vi "Periodic Tasks.vi"() -> ()   [LabVIEW 2011]
doc: "This VI runs in parallel to other tasks. It can contain as many user-defined periodic loops as you need. These can carry out PID or other sorts of timed response."
uses:
  <vilib>/Rock Robotics/SystemInterfaces/Utilities/FPGA_UtilitiesLED Source.ctl
  <vilib>/Rock Robotics/SystemInterfaces/Utilities/FPGA_UtilitiesLED State.ctl
  Robot Global Data.vi
  <vilib>/Rock Robotics/WPI/Relay/WPI_RelayValue.ctl
  <vilib>/addons/control/pid/NI_PID_pid.lvlib
  <vilib>/addons/control/pid/pid.llb/PID (DBL).vi
panel:
  out "Waveform Chart 2":dynamicdata(graph)
  in  "PID gains 2":T1={"proportional gain (Kc)"=1.0, "integral time (Ti, min)"=0.01, "derivative time (Td, min)"=0.0} {"derivative time (Td, min)" format="%.3f"; "integral time (Ti, min)" format="%.3f"; "proportional gain (Kc)" format="%.3f"}
  in  "Volts per degree":dbl=0.0166666666666667
  in  "-1/1 per degree":dbl=0.05
  in  "Home Speed 2":dbl=1.0
  in  "PID Enable 2":bool
  in  "lower limit 2":dbl=0.85
  in  "upper limit 2":dbl=4.5
  out "Whole Loop Timer":u32
  out "Heading 2":u16
  out "Angular Rate":dbl
  out "Angle":dbl
  out "Direction":bool
  out "Distance":dbl
  # "Speed to move to home"
  # "Target Tracking"
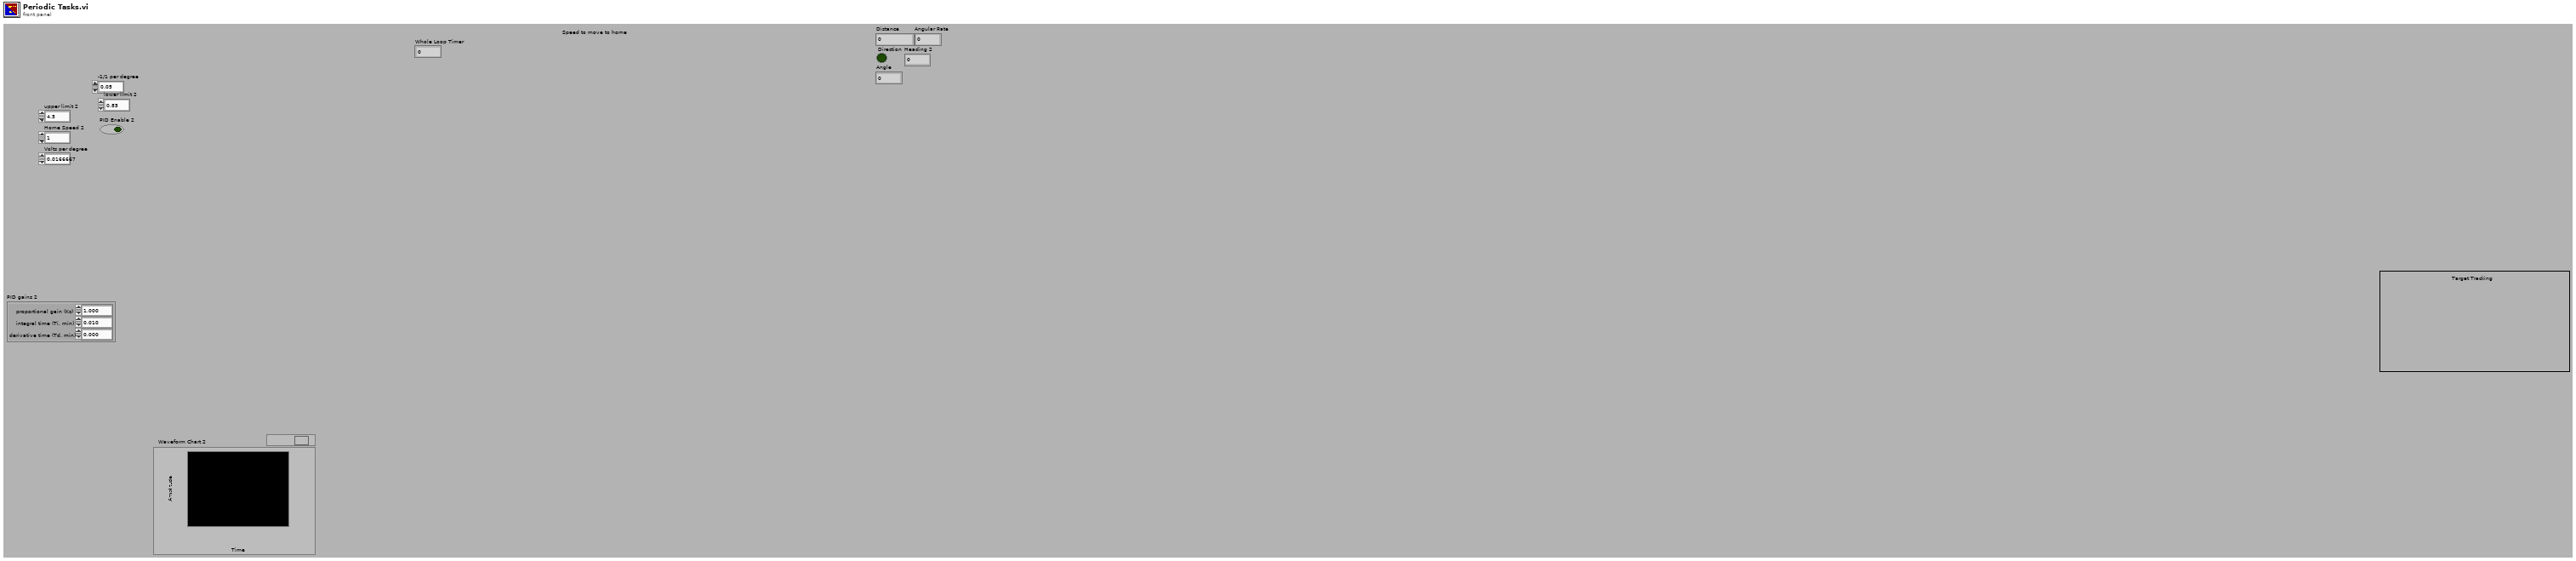
[diagram p1: front panel]
types:
  T1 = cluster{"proportional gain (Kc)":dbl, "integral time (Ti, min)":dbl, "derivative time (Td, min)":dbl}
  T2 = typedef "WPI_RelayValue.ctl" = enum16{"Off", "On", "Forward", "Reverse"}
  T3 = typedef "WPI_AnalogChannelDevRef.ctl" = cluster{"DevStatus":errorcluster, "Analog Module":T4, "Analog Channel":T5}
  T4 = typedef "FPGA_TypedefAnalogModule.ctl" = enum16{"Analog Module 1", "Analog Module 2"}
  T5 = typedef "FPGA_AIChannel.ctl" = enum8{"AI 1", "AI 2", "AI 3", "AI 4", "AI 5", "AI 6", "AI 7", "AI 8", "Invalid"}
  T6 = typedef "WPI_I2CDevRef.ctl" = cluster{"DevStatus":errorcluster, "Digital Module":T7, "Device Address":u8}
  T7 = typedef "FPGA_TypedefDigitalModule.ctl" = enum16{"Digital Module 1", "Digital Module 2"}
  T8 = cluster{"Driver Station Digital Output (1-8)[0]":bool, "Driver Station Digital Output (1-8)[1]":bool, "Driver Station Digital Output (1-8)[2]":bool, "Driver Station Digital Output (1-8)[3]":bool, "Driver Station Digital Output (1-8)[4]":bool, "Driver Station Digital Output (1-8)[5]":bool, "Driver Station Digital Output (1-8)[6]":bool, "Driver Station Digital Output (1-8)[7]":bool, "Driver Station Digital Output (1-8)[8]":bool}
  T9 = typedef "WPI_EncoderDevRef.ctl" = cluster{"DevStatus":errorcluster, "EncoderIndex":T10, "CounterIndex":T11, "DistancePerCount":dbl, "Decoding Type":T12}
  T10 = typedef "FPGA_EncoderIdx.ctl" = enum8{"Enc 0", "Enc 1", "Enc 2", "Enc 3", "Invalid"}
  T11 = typedef "FPGA_CounterCtrSystemIndex.ctl" = enum8{"Ctr 0", "Ctr 1", "Ctr 2", "Ctr 3", "Ctr 4", "Ctr 5", "Ctr 6", "Ctr 7", "Invalid"}
  T12 = typedef "WPI_EncoderType.ctl" = enum16{"1x", "2x", "4x"}
  T13 = typedef "WPI_GyroDevRef.ctl" = cluster{"DevStatus":errorcluster, "Analog Module":T4, "Analog Channel":T5, "Offset":dbl, "Gain (VoltsPerDegree/Second)":dbl}
  T14 = typedef "WPI_RelayDevRef.ctl" = cluster{"DevStatus":errorcluster, "Relay Channel":T15, "Digital Module":T7, "Relay Direction":T16}
  T15 = typedef "FPGA_DIORelayChannel.ctl" = enum8{"Relay 1", "Relay 2", "Relay 3", "Relay 4", "Relay 5", "Relay 6", "Relay 7", "Relay 8", "Invalid"}
  T16 = typedef "WPI_RelayDirection.ctl" = enum16{"Both directions", "Forward only", "Reverse only"}
  T17 = typedef "FPGA_UtilitiesLED State.ctl" = enum16{"Off", "On", "Toggle"}
  T18 = typedef "FPGA_UtilitiesLED Source.ctl" = enum16{"User LED", "FPGA LED"}
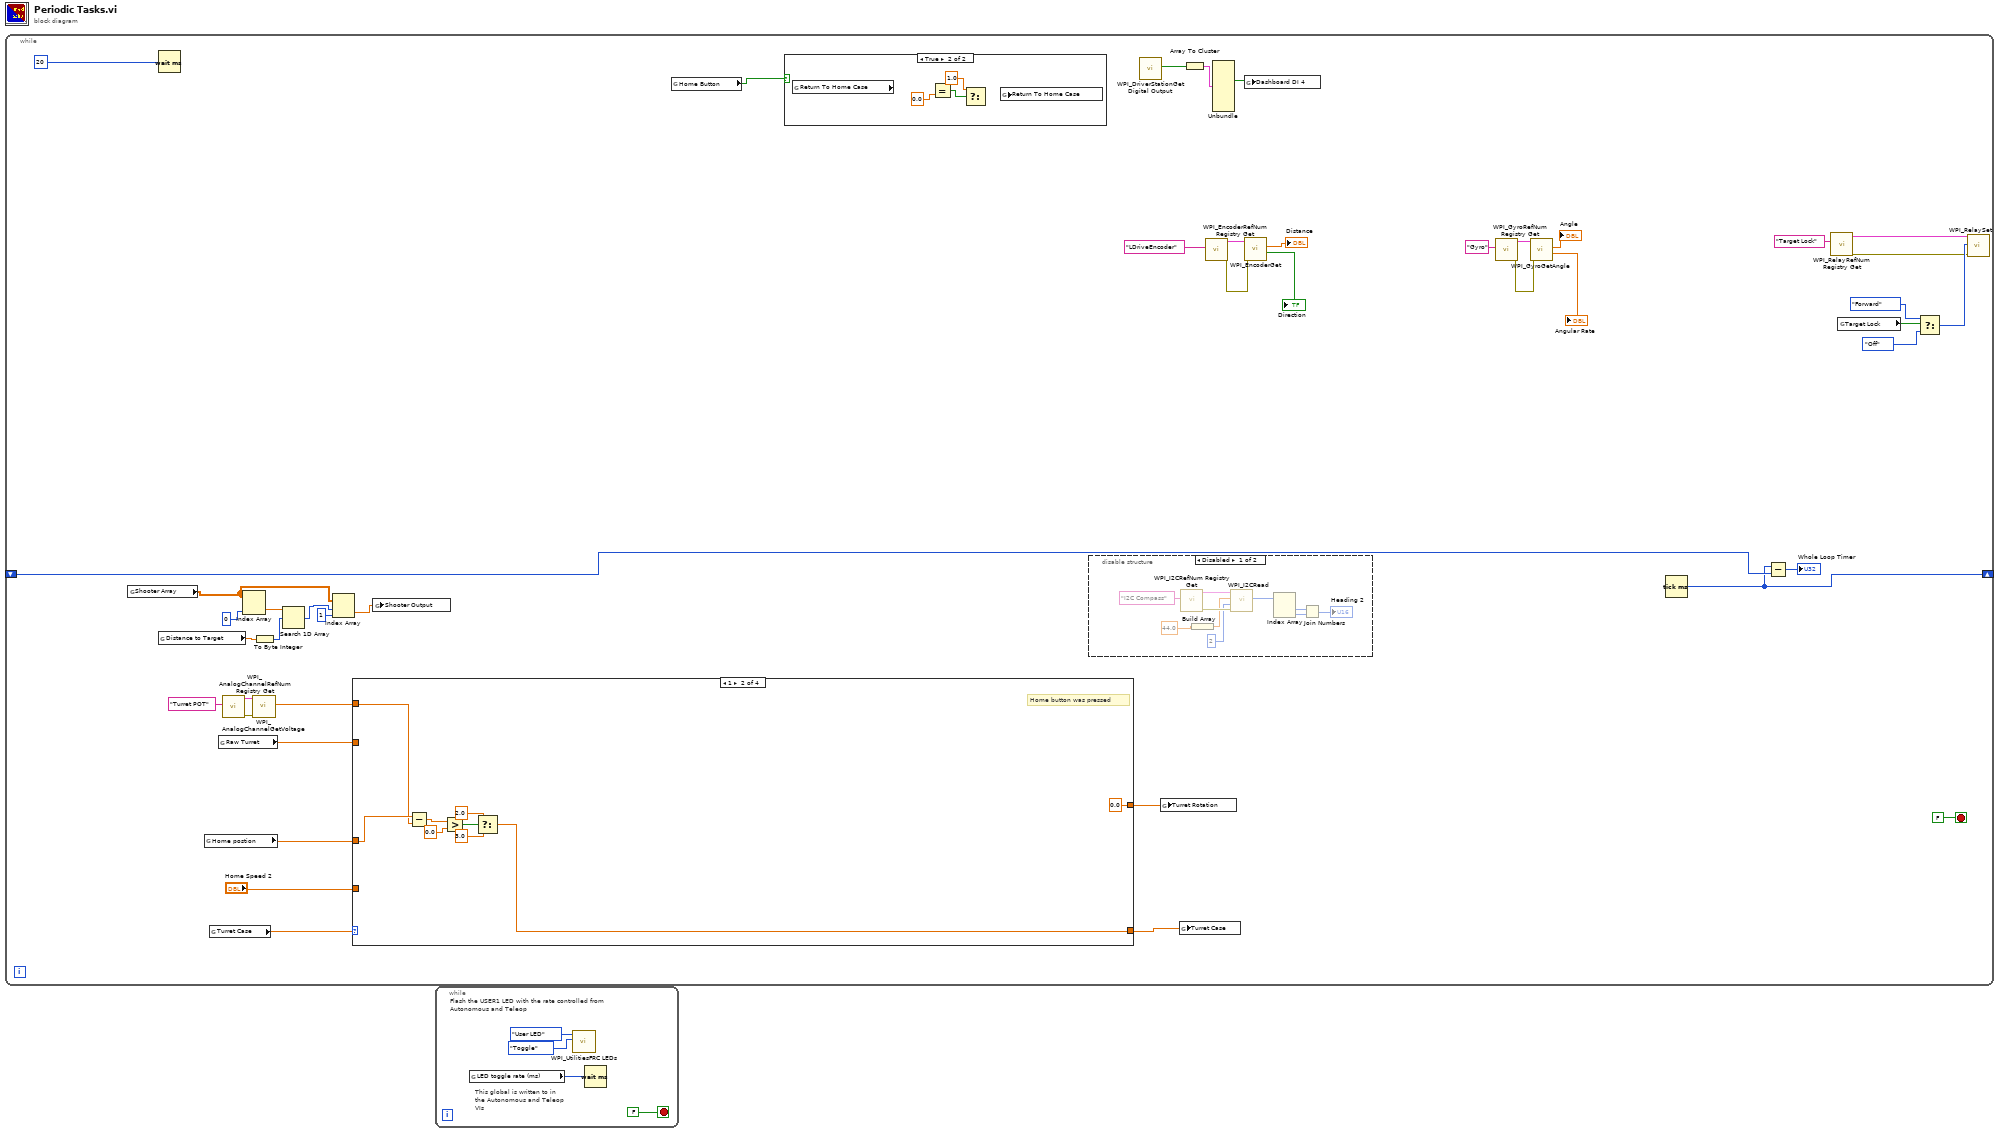
[diagram p0: block diagram]
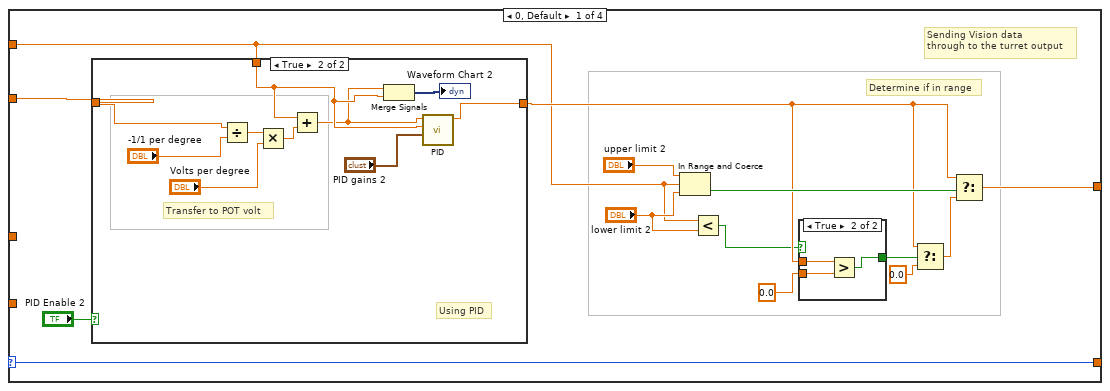
[diagram p2: hidden frame]
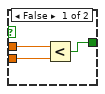
[diagram p3: hidden frame]
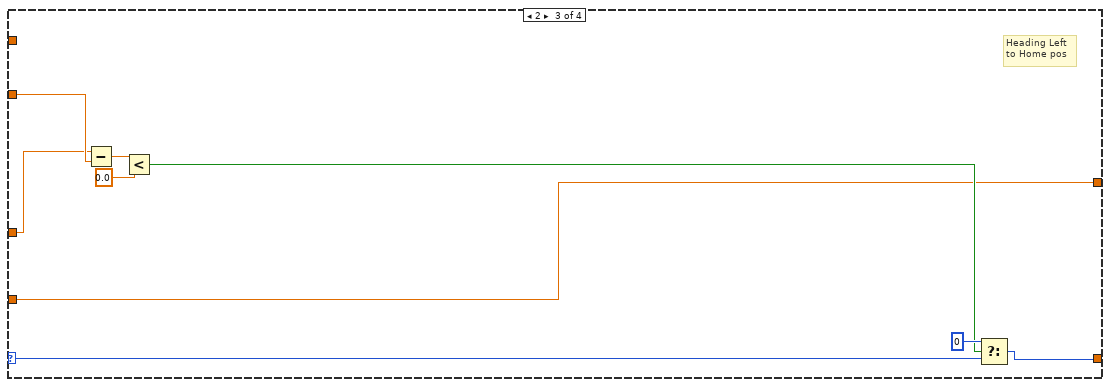
[diagram p5: hidden frame]
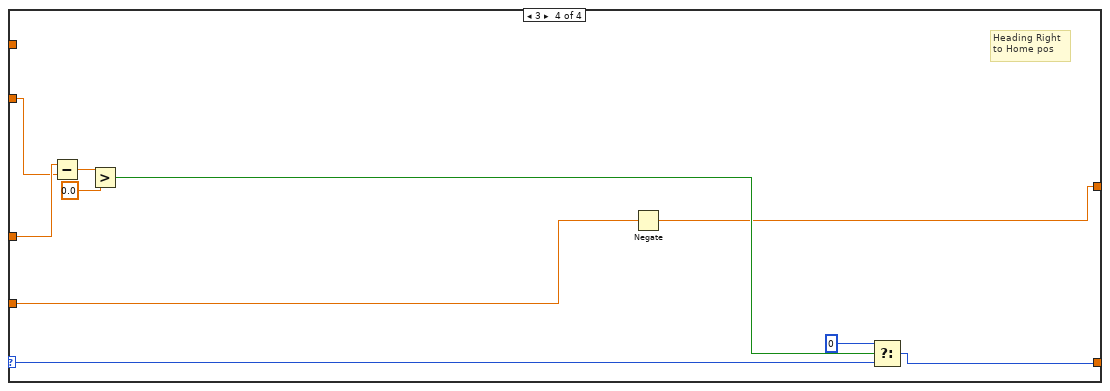
[diagram p6: hidden frame]
diagram:
  n1 = while {
    shift-right: [w12] -> _
    shift-left: _ -> [w13]
    stop <- FALSE stop-if-true
    n2 = global read "Robot Global Data.vi" "Shooter Array"() -> (w15:dbl[][])
    n3 = Wait (ms)(milliseconds to wait=u32 20) -> ()  [unwired: 1 out]
    n4 = global read "Robot Global Data.vi" "Distance to Target"() -> (w17:dbl)
    n5 = global read "Robot Global Data.vi" "Home postion"() -> (w3:dbl)
    n6 = global read "Robot Global Data.vi" "Turret Case"() -> (w10:dbl)
    n7 = global read "Robot Global Data.vi" "Raw Turret"() -> (w5:dbl)
    n8 = call <vilib>:"WPI_AnalogChannelRefNum Registry Get.vi"("refnum name"="Turret POT") -> ("error out"=w9:errorcluster, "AIDeviceRef"=w8:T3)  [unwired: 9 in]
    n9 = Index Array(array=w15, index (col)=0 ("disabled index (col)")) -> (element=w20:dbl[])  [unwired: 1 in]
    n10 = call <vilib>:"WPI_AnalogChannelGetVoltage.vi"("error in (no error)"=w9, "AIDeviceRef"=w8) -> ("Voltage"=w6:dbl)  [unwired: 7 in, 2 out]
    n11 = To Byte Integer(number=w17) -> (8bit integer=w16:i8)
    n12 = Search 1D Array(1D array=w20, element=w16) -> (index of element=w18:i32)  [unwired: 1 in]
    n13 = Index Array(array=w15, index (row)=w18, index (col)=1) -> (element=w14:dbl)
    n14 = case shown="1" w10 {
      selector: w10 -> [w46 _ w88 w98]
      tunnel: w6 -> [w45 w78 _ _]
      tunnel: w5 -> [w55 _ w91 w100]
      tunnel: [w47 0.0 ("Home Speed 2") w85 w94] -> w4
      tunnel: w3 -> [_ w79 w90 w101]
      tunnel: [w46 w77 w87 w97] -> w2
      tunnel: "Home Speed 2" -> [_ _ w85 w95]
      frame 0, Default {
        # "Determine if in range"
        # "Sending Vision data\nthrough to the turret output"
        n15 = case shown="True" "PID Enable 2" {
          tunnel: w55 -> [w65 w74]
          tunnel: [w65 w69] -> w51
          tunnel: w45 -> [_ w67]
          frame False {
            # "Using my logic"
          }
          frame True {
            # "Transfer to POT volt"
            # "Using PID"
            n16 = Divide(x=w74, y="-1/1 per degree") -> (x/y=w73:dbl)
            n17 = Multiply(x=w73, y="Volts per degree") -> (x*y=w71:dbl)
            n18 = Add(x=w67, y=w71) -> (x+y=w66:dbl)
            n19 = Merge Signals(w66, w67) -> (→"Waveform Chart 2":dynamicdata)
            n20 = call-poly <vilib>:"PID.vi"("PID gains"="PID gains 2", "process variable"=w67, "setpoint"=w66) -> ("output"=w69:dbl)  [unwired: 7 in, 1 out]
          }
        }
        n21 = In Range and Coerce(upper limit="upper limit 2", x=w45, lower limit="lower limit 2") -> (In Range?=w56:bool)  [unwired: 1 out]
        n22 = Less?(x=w45, y="lower limit 2") -> (x < y?=w48:bool)
        n23 = case shown="True" w48 {
          tunnel: 0.0 -> [w60 w64]
          tunnel: [w59 w63] -> w52
          tunnel: w51 -> [w61 w62]
          frame False {
            n24 = Less?(x=w61, y=w60) -> (x < y?=w59:bool)
          }
          frame True {
            n25 = Greater?(x=w62, y=w64) -> (0:w63:bool)
          }
        }
        n26 = Select(t=w51, s=w52, f=0.0) -> (s? t:f=w50:dbl)
        n27 = Select(t=w51, s=w56, f=w50) -> (s? t:f=w47:dbl)
      }
      frame 1 {
        # "Home button was pressed"
        n28 = Subtract(x=w79, y=w78) -> (x-y=w80:dbl)
        n29 = Greater?(x=w80, y=0.0) -> (0:w82:bool)
        n30 = Select(t=2.0, s=w82, f=3.0) -> (s? t:f=w77:dbl)
      }
      frame 2 {
        # "Heading Left\nto Home pos"
        n31 = Subtract(x=w90, y=w91) -> (x-y=w92:dbl)
        n32 = Less?(x=w92, y=0.0) -> (x < y?=w86:bool)
        n33 = Select(t=0, s=w86, f=w88) -> (s? t:f=w87:i32)
      }
      frame 3 {
        # "Heading Right\nto Home pos"
        n34 = Subtract(x=w101, y=w100) -> (x-y=w102:dbl)
        n35 = Greater?(x=w102, y=0.0) -> (0:w96:bool)
        n36 = Negate(x=w95) -> (-x=w94:dbl)
        n37 = Select(t=0, s=w96, f=w98) -> (s? t:f=w97:i32)
      }
    }
    n38 = global write "Robot Global Data.vi" "Shooter Output"(w14) -> ()
    n39 = global read "Robot Global Data.vi" "Home Button"() -> (w33:bool)
    n40 = case shown="True" w33 {
      frame False {
      }
      frame True {
        n41 = global read "Robot Global Data.vi" "Return To Home Case"() -> ()  [unwired: 1 out]
        n42 = Equal?(y=0.0) -> (x = y?=w115:bool)  [unwired: 1 in]
        n43 = Select(t=1.0, s=w115) -> ()  [unwired: 1 in, 1 out]
        n44 = global read "Robot Global Data.vi" "Return To Home Case"() -> ()  [unwired: 1 in]
      }
    }
    n45 = disable-structure shown="Disabled" {
      frame Disabled {
        n46 = call <vilib>:"WPI_I2CRefNum Registry Get.vi"("refnum name"="I2C Compass") -> ("error out"=w113:errorcluster, "I2CDevRef"=w112:T6)  [unwired: 9 in]
        n47 = Build Array(44.0 ("element")) -> (w106:dbl[])
        n48 = call <vilib>:"WPI_I2CRead.vi"("error in (no error)"=w113, "I2CBytesToRead"=u8 2, "I2CRegister"=w106, "I2CDevRef"=w112) -> ("Data Out"=w110:u8[])  [unwired: 5 in, 2 out]
        n49 = Index Array(array=w110) -> (element #1=w108:u8, element #2=w109:u8)  [unwired: 2 in]
        n50 = Join Numbers(hi=w108, lo=w109) -> ((hi.lo)=→"Heading 2":u16)
      }
      frame Enabled {
      }
    }
    n51 = call <vilib>:"WPI_DriverStationGet Digital Output.vi"() -> ("Driver Station Digital Output (1-8)"=w44:bool[])  [unwired: 10 in, 1 out]
    n52 = global write "Robot Global Data.vi" "Turret Rotation"(w4) -> ()
    n53 = global write "Robot Global Data.vi" "Turret Case"(w2) -> ()
    n54 = Array To Cluster(array=w44) -> (cluster=w43:T8)
    n55 = call <vilib>:"WPI_EncoderRefNum Registry Get.vi"("refnum name"="LDriveEncoder") -> ("error out"=w28:errorcluster, "EncoderDevRef"=w29:T9)  [unwired: 9 in]
    n56 = Unbundle(w43) -> ("Driver Station Digital Output (1-8)[3]"=w42:bool)  [unwired: 8 out]
    n57 = global write "Robot Global Data.vi" "Dashboard DI 4"(w42) -> ()
    n58 = call <vilib>:"WPI_EncoderGet.vi"("error in (no error)"=w28, "EncoderDevRef"=w29) -> ("Direction"=→"Direction":bool, "Distance"=→"Distance":dbl)  [unwired: 4 in, 4 out]
    n59 = call <vilib>:"WPI_GyroRefNum Registry Get.vi"("refnum name"="Gyro") -> ("error out"=w25:errorcluster, "GyroDevRef"=w26:T13)  [unwired: 9 in]
    n60 = call <vilib>:"WPI_GyroGetAngle.vi"("error in (no error)"=w25, "GyroDevRef"=w26) -> ("Angular Rate"=→"Angular Rate":dbl, "Angle"=→"Angle":dbl)  [unwired: 6 in, 2 out]
    n61 = Tick Count (ms)() -> (millisecond timer value=w12:u32)
    n62 = Subtract(x=w12, y=w13) -> (x-y=→"Whole Loop Timer":u32)
    n63 = call <vilib>:"WPI_RelayRefNum Registry Get.vi"("refnum name"="Target Lock") -> ("error out"=w35:errorcluster, "RelayDevRef"=w36:T14)  [unwired: 9 in]
    n64 = global read "Robot Global Data.vi" "Target Lock"() -> (w41:bool)
    n65 = Select(t=WPI_RelayValue."Forward" ("RelayValue"), s=w41, f=WPI_RelayValue."Off" ("RelayValue")) -> (s? t:f=w38:T2)
    n66 = call <vilib>:"WPI_RelaySet.vi"("error in (no error)"=w35, "RelayValue"=w38, "RelayDevRef"=w36) -> ()  [unwired: 7 in, 2 out]
  }
  n67 = while {
    stop <- FALSE stop-if-true
    # "This global is written to in the Autonomous and Teleop VIs"
    # "Flash the USER1 LED with the rate controlled from Autonomous and Teleop"
    n68 = global read "Robot Global Data.vi" "LED toggle rate (ms)"() -> (w117:u32)
    n69 = call <vilib>:"WPI_UtilitiesFRC LEDs.vi"("State"=FPGA_UtilitiesLED_State."Toggle", "LED Type"=FPGA_UtilitiesLED_Source."User LED") -> ()  [unwired: 1 in, 9 out]
    n70 = Wait (ms)(milliseconds to wait=w117) -> ()  [unwired: 1 out]
  }
